vi "CSM - Generate User Global Log.vi"(6 "From Who":string, 7 "Place (\"\" to Use VI's Name)":string, 8 "Error In":errorcluster caption="error in (no error)", 10 "Arguments":string, 11 "Log":string) -> (0 "error out":errorcluster)   [LabVIEW 2017, in "Communicable State Machine.lvlib"]
doc: "Generates a custom user log for scenarios such as debugging. When the input parameters of this VI contain error information, CSM - Global Log Error Handler VI is called to record the error information.\n\n-- <b>Controls</b> --\n\n- <b>Log</b>: Event name.\n- <b>Arguments</b>: Event arguments.\n- <b>From Who</b>: Source.\n- <b>ModuleName</b>: Module name.\n- <b>Place (\"\" to Use VI's Name)</b>: Location where the error occurred. The default is the name of the VI."
uses:
  Communicable State Machine.lvlib
  _Support/Typedef/_CSM_GlobalLog_MSG.ctl
  _Support/Typedef/_CSM_Response Source Message.ctl
  _Support/Typedef/_CSM_GlobalLog_MSG_TYPE.ctl
  _Support/GlobalEvent/LogFilter/LogFilter.lvclass
  CSM - Make String Arguments Safe.vi
  CSM - Keywords.vi
  _Support/GlobalEvent/LogFilter/LogFilter - Check.vi
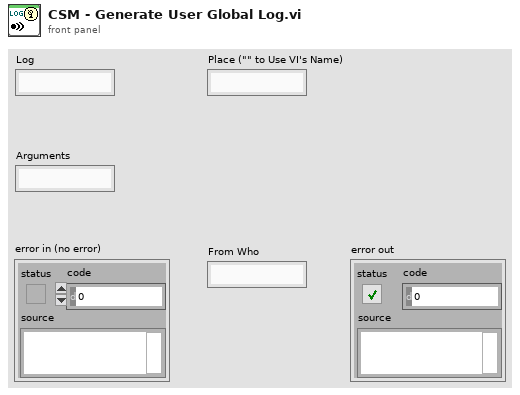
[diagram p1: front panel]
types:
  T1 = typedef "Communicable State Machine.lvlib/GEvt-Refs.ctl" = cluster{"Event":refnum<user-event>, "Queues":refnum<queue>[], "Valid":bool}
  T2 = typedef "Communicable State Machine.lvlib/_CSM_GlobalLog_MSG_TYPE.ctl" = enum16{"User Log", "State Change", "Status", "Interrupt", "Register", "Unregister", "Error Log", "Module Created", "Module Destroyed", "Async Message", "No-Rep Async Message", "Sync Message"}
  T3 = typedef "Communicable State Machine.lvlib/_CSM_GlobalLog_MSG.ctl" = cluster{"Name (\"\" to Use UUID)":string, "Current State":string, "Arguments":string, "Source Message":T4, "Source Module":string, "Complete(T)/Start(F)":bool, "LogType":T2, "Time Stamp":timestamp}
  T4 = typedef "Communicable State Machine.lvlib/_CSM_Response Source Message.ctl" = cluster{"‘State":string, "’Arguments":string, "’Error":errorcluster}
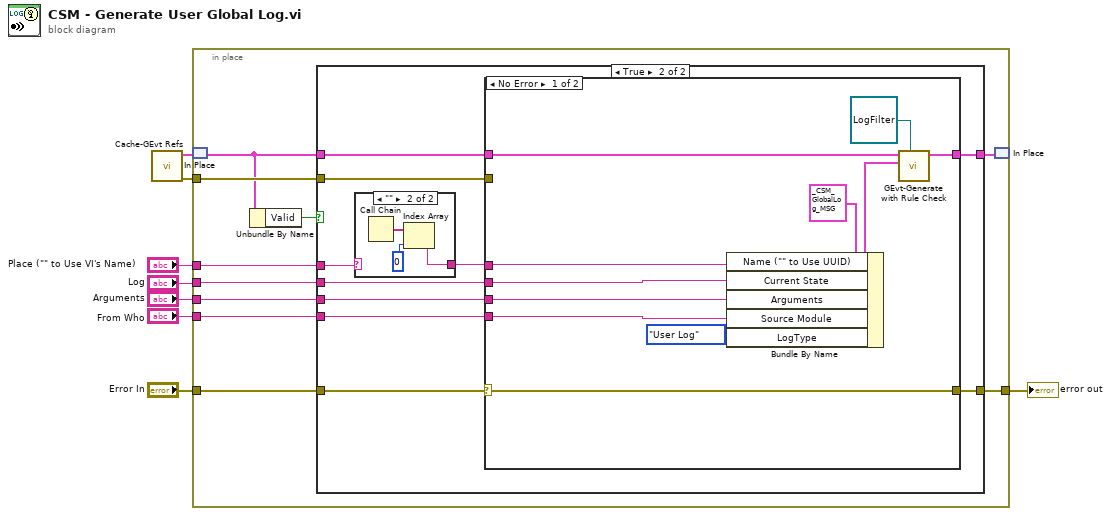
[diagram p0: block diagram]
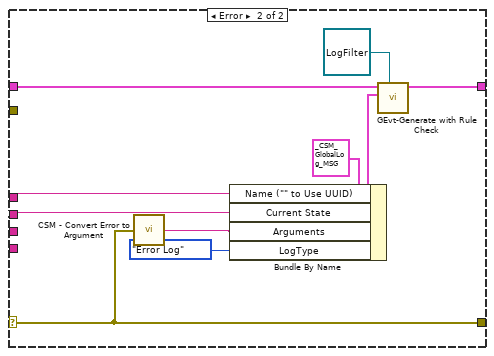
[diagram p4: hidden frame]
diagram:
  n1 = call "Cache-GEvt Refs.vi"() -> ("error out"=w1:errorcluster, "CSM Global Log Ref"=w2:T1)  [unwired: 10 in]
  n2 = in-place {
    in-place-border: "Place (\"\" to Use VI's Name)" -> [w17]
    in-place-border: "Log" -> [w16]
    in-place-border: "Arguments" -> [w15]
    in-place-border: w1 -> [w14]
    in-place-border: [w13] -> w8
    in-place-border: "From Who" -> [w12]
    in-place-border: "Error In" -> [w11]
    n3 = in-place-match #1(w2) -> (w10:T1)
    n4 = Unbundle By Name(w10) -> ("Valid"=w9:bool)
    n5 = case shown="True" w9 {
      tunnel: w10 -> [w20 w30]
      tunnel: w17 -> [_ w22]
      tunnel: [w20 w29] -> w18
      tunnel: w16 -> [_ w28]
      tunnel: w15 -> [_ w27]
      tunnel: w14 -> [w19 w26]
      tunnel: [w19 w25] -> w13
      tunnel: w12 -> [_ w24]
      tunnel: w11 -> [_ w23]
      frame False {
      }
      frame True {
        n6 = case shown="\"\"" w22 {
          selector: w22 -> [w31 _]
          tunnel: [w31 w32] -> w21
          frame Default {
          }
          frame "" {
            n7 = Call Chain() -> (call chain=w33:string[])
            n8 = Index Array(array=w33, index=0 ("Index")) -> (element=w32:string)
          }
        }
        n9 = case shown="No Error" w23 {
          selector: w23 -> [w37 w53]
          tunnel: w30 -> [w45 w55]
          tunnel: [w42 w54] -> w29
          tunnel: w28 -> [w41 w48]
          tunnel: w27 -> [w40 _]
          tunnel: w26 -> [_ _]
          tunnel: [w37 w53] -> w25
          tunnel: w24 -> [w38 _]
          tunnel: w21 -> [w36 w47]
          frame No Error {
            n10 = Bundle By Name(cluster=T3 {"Name (\"\" to Use UUID)"="", "Current State"="", "Arguments"="", "Source Message"={"‘State"="", "’Arguments"="", "’Error"={"status"=FALSE, "code"=0, "source"=""}}, "Source Module"="", "Complete(T)/Start(F)"=FALSE, "LogType"=enum."User Log", "Time Stamp"=timestamp(0 s since 1904-01-01)} ("event data"), "Name (\"\" to Use UUID)"=w36, "Current State"=w41, "Arguments"=w40, "Source Module"=w38, "LogType"=_CSM_GlobalLog_MSG_TYPE."User Log" ("Type")) -> (w43:T3)
            n11 = call "GEvt-Generate with Rule Check.vi"("LogFilter In"=refnum<class "LogFilter.lvclass"> refnum ("LogFilter in"), "Event Data"=w43, "CSM Global Log Event In"=w45) -> ("CSM Global Log Event Out"=w42:T1)  [unwired: 8 in]
          }
          frame Error {
            n12 = call "CSM - Convert Error to Argument.vi"("Error"=w53) -> ("Argument"=w49:string)  [unwired: 4 in]
            n13 = Bundle By Name(cluster=T3 {"Name (\"\" to Use UUID)"="", "Current State"="", "Arguments"="", "Source Message"={"‘State"="", "’Arguments"="", "’Error"={"status"=FALSE, "code"=0, "source"=""}}, "Source Module"="", "Complete(T)/Start(F)"=FALSE, "LogType"=enum."User Log", "Time Stamp"=timestamp(0 s since 1904-01-01)} ("event data"), "Name (\"\" to Use UUID)"=w47, "Current State"=w48, "Arguments"=w49, "LogType"=_CSM_GlobalLog_MSG_TYPE."Error Log" ("Type")) -> (w51:T3)
            n14 = call "GEvt-Generate with Rule Check.vi"("LogFilter In"=refnum<class "LogFilter.lvclass"> refnum ("LogFilter in"), "Event Data"=w51, "CSM Global Log Event In"=w55) -> ("CSM Global Log Event Out"=w54:T1)  [unwired: 8 in]
          }
        }
      }
    }
    n15 = in-place-match #1(w18) -> ()  [unwired: 1 out]
  }
  "error out" <- w8
